vi "SC2 Host.vi"() -> ()   [LabVIEW 2015]
uses:
  SC2 states.ctl
  Interface states.ctl
panel:
  out "Change Complete?":bool
  out "Motor status":bool
  out "Current Sample":u8
  in  "Random Change":bool
  in  "stop":bool
  out "error out":errorcluster
  in  "error in (no error)":errorcluster
  in  "Encoder Offset":i16=-1021
  in  "Requested Sample":u8
  out "SC2 State Control":T1=enum."wait"
  out "Raw Encoder":bool[](array[boolean])
  out "Converted Encoder":bool[](array[boolean])
  out "Encoder Position":i32
  out "Motor Done?":bool
  in  "Start Sample Change":bool
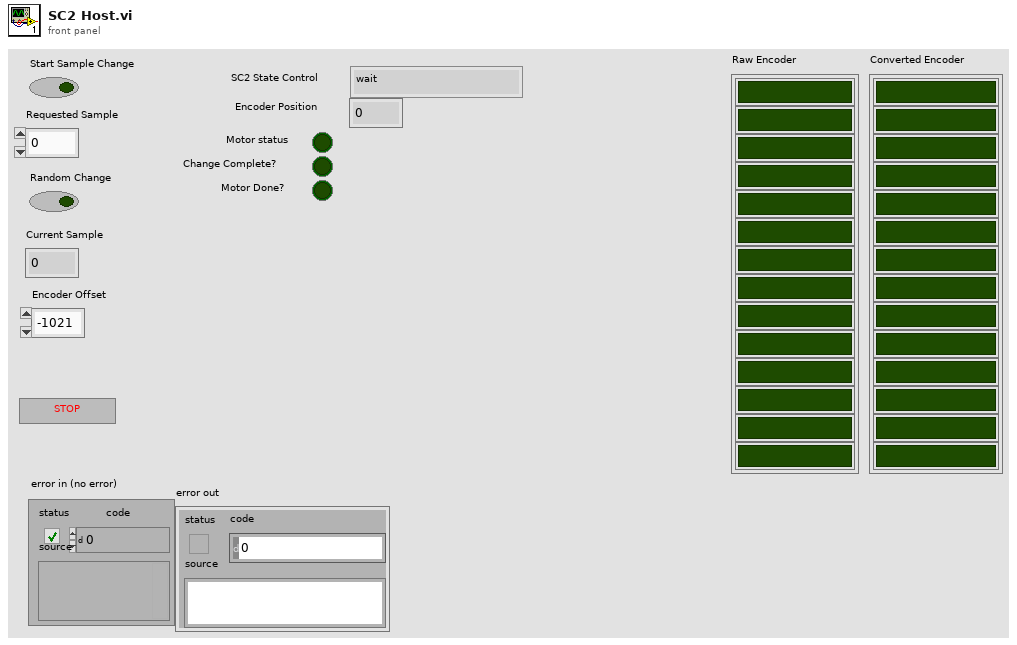
[diagram p1: front panel]
types:
  T1 = typedef "SC2 states.ctl" = enum16{"initialize", "wait", "check position", "rotate wheel", "rotate complete"}
  T2 = typedef "Interface states.ctl" = enum16{"Initialization", "Wait", "start wheel change", "Shutdown"}
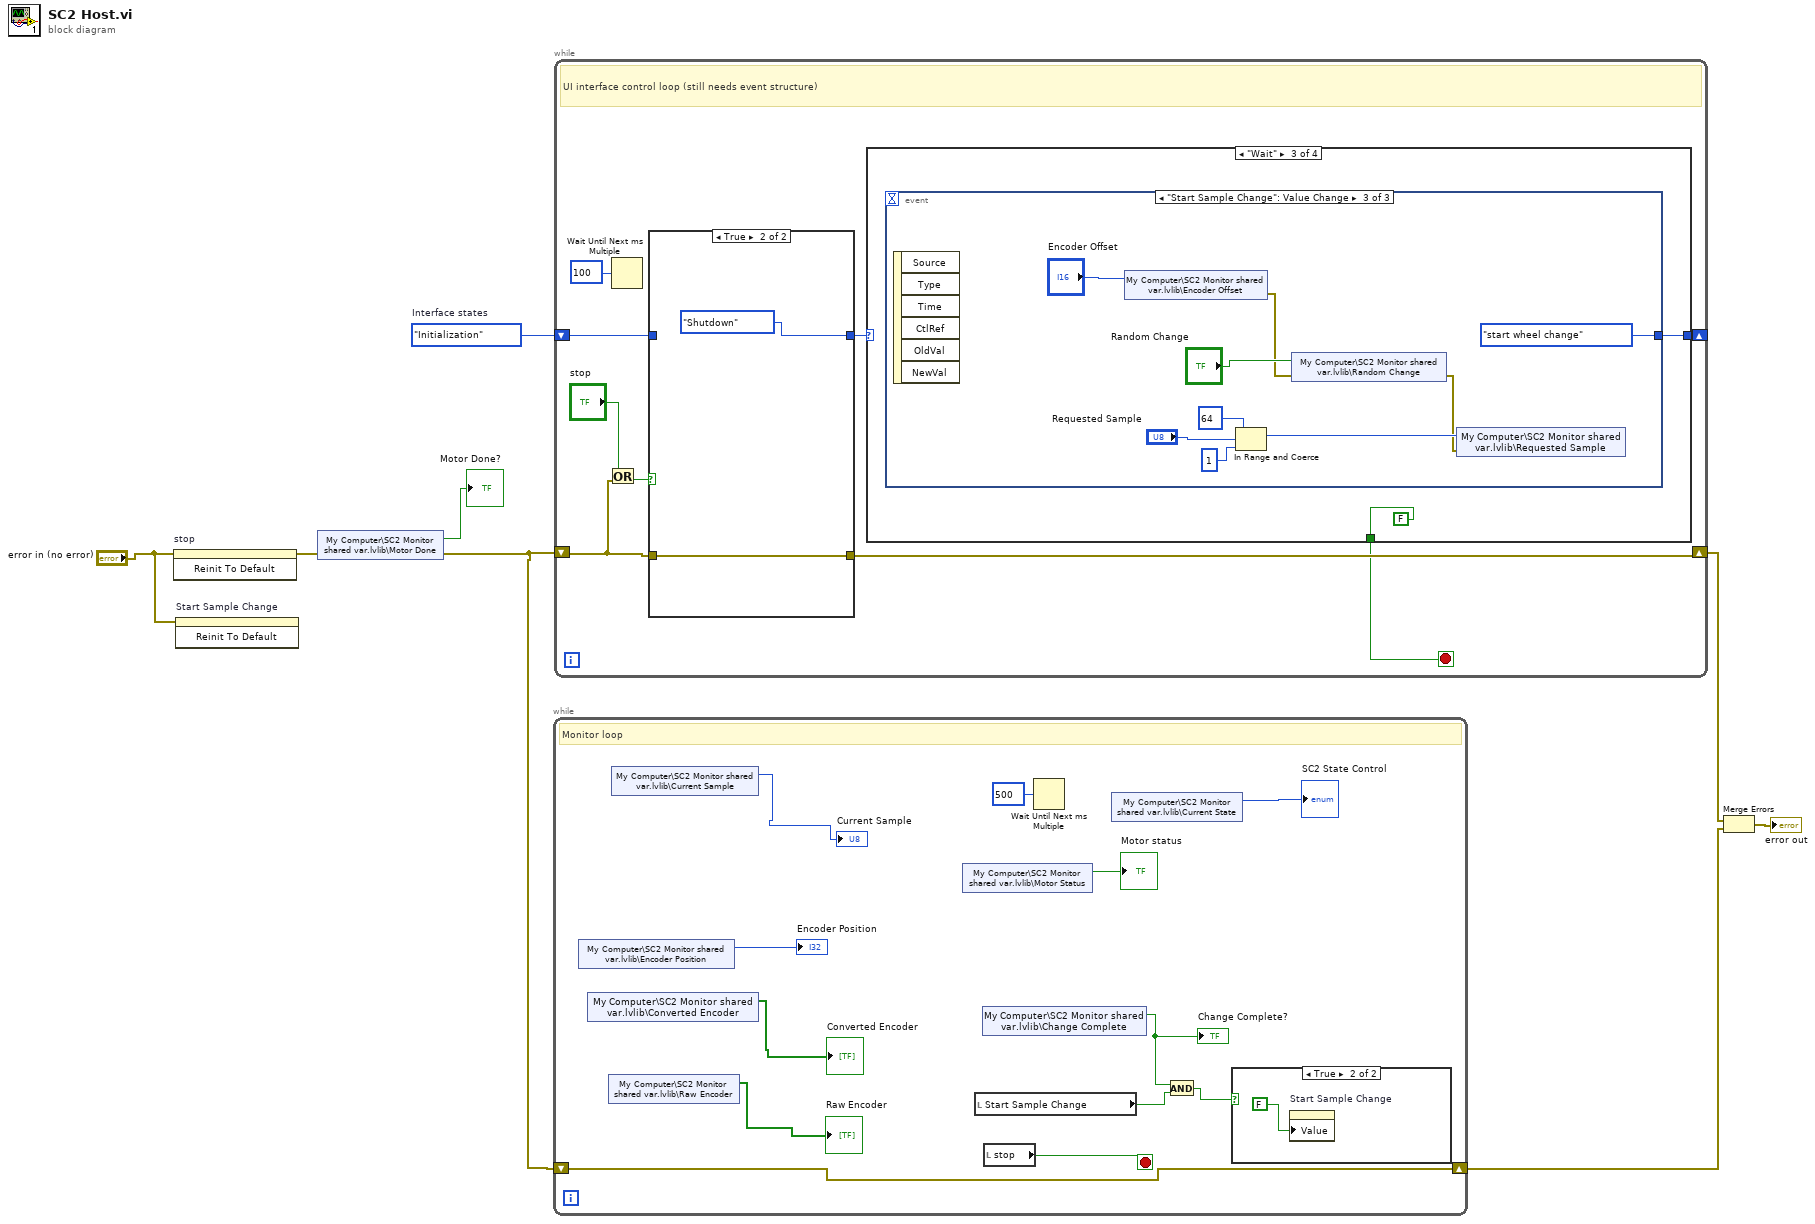
[diagram p0: block diagram]
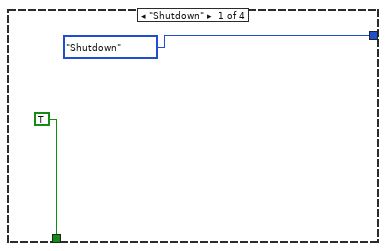
[diagram p4: hidden frame]
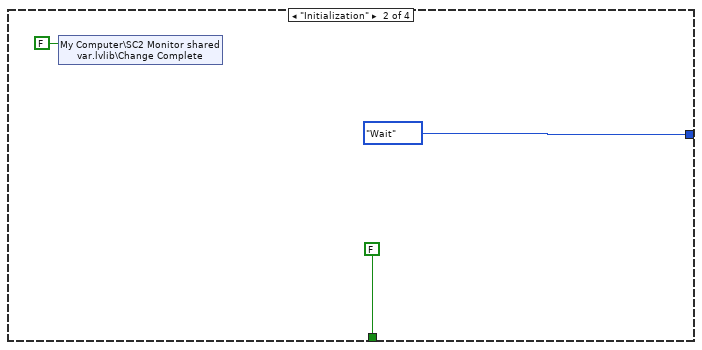
[diagram p5: hidden frame]
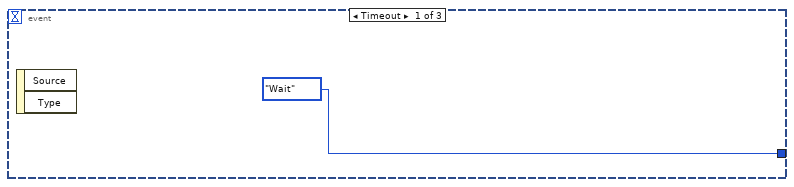
[diagram p6: hidden frame]
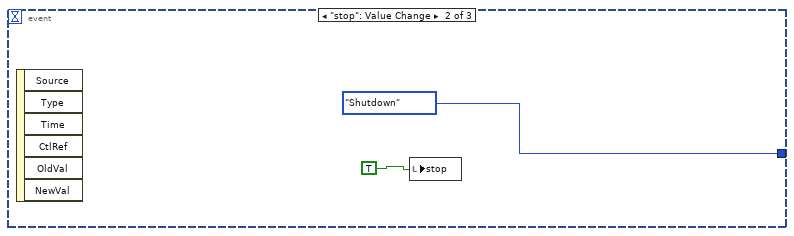
[diagram p7: hidden frame]
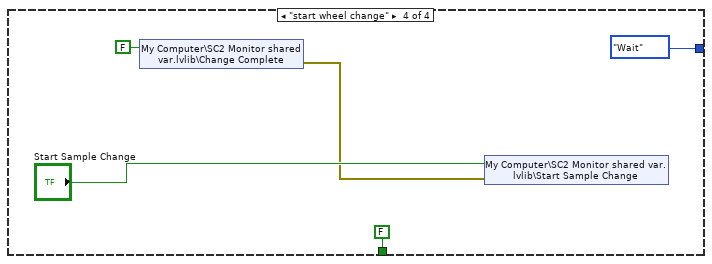
[diagram p8: hidden frame]
diagram:
  w3 = Interface_states."Initialization"  # Interface states
  n1 = invoke on="stop" class="Bool (strict)" method="Reinit To Default"(error in="error in (no error)") -> (error out=w1:errorcluster)  [unwired: 2 in, 2 out]
  n2 = invoke on="Start Sample Change" class="Bool (strict)" method="Reinit To Default"(error in="error in (no error)") -> ()  [unwired: 2 in, 3 out]
  n3 = shared-variable "My Computer\\SC2 Monitor shared var.lvlib\\Motor Done"(error in=w1) -> (→"Motor Done?":bool, error out=w4:errorcluster)
  n4 = while {
    shift-right: [w19] -> w6
    shift-left: w4 -> [w19]
    stop <- w18 stop-if-true
    # "Monitor loop"
    n5 = shared-variable "My Computer\\SC2 Monitor shared var.lvlib\\Encoder Position"() -> (→"Encoder Position":i32)  [unwired: 1 in, 1 out]
    n6 = shared-variable "My Computer\\SC2 Monitor shared var.lvlib\\Converted Encoder"() -> (→"Converted Encoder":bool[])  [unwired: 1 in, 1 out]
    n7 = shared-variable "My Computer\\SC2 Monitor shared var.lvlib\\Raw Encoder"() -> (→"Raw Encoder":bool[])  [unwired: 1 in, 1 out]
    n8 = shared-variable "My Computer\\SC2 Monitor shared var.lvlib\\Current Sample"() -> (→"Current Sample":u8)  [unwired: 1 in, 1 out]
    n9 = shared-variable "My Computer\\SC2 Monitor shared var.lvlib\\Motor Status"() -> (→"Motor status":bool)  [unwired: 1 in, 1 out]
    n10 = local read "Start Sample Change"() -> (w16:bool)
    n11 = shared-variable "My Computer\\SC2 Monitor shared var.lvlib\\Change Complete"() -> (w12:bool)  [unwired: 1 in, 1 out]
    "Change Complete?" <- w12
    n12 = local read "stop"() -> (w18:bool)
    n13 = Wait Until Next ms Multiple(millisecond multiple=u32 500) -> ()  [unwired: 1 out]
    n14 = shared-variable "My Computer\\SC2 Monitor shared var.lvlib\\Current State"() -> (→"SC2 State Control":u16)  [unwired: 1 in, 1 out]
    n15 = And(x=w12, y=w16) -> (x .and. y?=w17:bool)
    n16 = case shown="True" w17 {
      frame False {
      }
      frame True {
        n17 = property on="Start Sample Change" class="Bool (strict)"("Value"=FALSE ("Start Sample Change")) -> ()  [unwired: 2 in, 2 out]
      }
    }
  }
  n18 = while {
    shift-right: [w27] -> w5
    shift-left: w4 -> [w23]
    shift-right: [w29] -> _
    shift-left: w3 -> [w25]
    stop <- w22 stop-if-true
    # "UI interface control loop (still needs event structure)"
    n19 = Or(x="stop", y=w23) -> (x .or. y?=w24:bool)
    n20 = Wait Until Next ms Multiple(millisecond multiple=u32 100) -> ()  [unwired: 1 out]
    n21 = case shown="True" w24 {
      tunnel: w23 -> [w32 w33]
      tunnel: [w32 w33] -> w27
      tunnel: [w31 Interface_states."Shutdown" ("Interface states")] -> w26
      tunnel: w25 -> [w31 _]
      frame False {
      }
      frame True {
      }
    }
    n22 = case shown="\"Wait\"" w26 {
      tunnel: [Interface_states."Shutdown" ("Interface states") Interface_states."Wait" ("Interface states") w40 Interface_states."Wait" ("Interface states")] -> w29
      tunnel: [TRUE FALSE FALSE FALSE] -> w22
      frame "Shutdown" {
      }
      frame "Initialization" {
        n23 = shared-variable "My Computer\\SC2 Monitor shared var.lvlib\\Change Complete"(FALSE ("SC2 Change Complete")) -> ()  [unwired: 1 in, 1 out]
      }
      frame "Wait" {
        n24 = event shown="[2] \"Start Sample Change\": Value Change" {
          selector: _ -> [_ _ _]
          dyn-events: _ -> [_ _ _]
          timeout: _ -> [_ _ _]
          tunnel: [Interface_states."Wait" ("Interface states") Interface_states."Shutdown" ("Interface states") Interface_states."start wheel change" ("Interface states")] -> w40
          event Timeout {
            n25 = event-data() -> ()  [unwired: 1 in, 2 out]
          }
          event "stop": Value Change {
            n26 = event-data() -> ()  [unwired: 1 in, 6 out]
            n27 = local write "stop"(TRUE ("stop")) -> ()
          }
          event "Start Sample Change": Value Change {
            n28 = event-data() -> ()  [unwired: 1 in, 6 out]
            n29 = shared-variable "My Computer\\SC2 Monitor shared var.lvlib\\Encoder Offset"("Encoder Offset") -> (error out=w45:errorcluster)  [unwired: 1 in]
            n30 = In Range and Coerce(upper limit=u8 64, x="Requested Sample", lower limit=u8 1) -> (coerced(x)=w51:u8)  [unwired: 1 out]
            n31 = shared-variable "My Computer\\SC2 Monitor shared var.lvlib\\Random Change"("Random Change", error in=w45) -> (error out=w47:errorcluster)
            n32 = shared-variable "My Computer\\SC2 Monitor shared var.lvlib\\Requested Sample"(w51, error in=w47) -> ()  [unwired: 1 out]
          }
        }
      }
      frame "start wheel change" {
        n33 = shared-variable "My Computer\\SC2 Monitor shared var.lvlib\\Change Complete"(FALSE ("SC2 Change Complete")) -> (error out=w54:errorcluster)  [unwired: 1 in]
        n34 = shared-variable "My Computer\\SC2 Monitor shared var.lvlib\\Start Sample Change"("Start Sample Change", error in=w54) -> ()  [unwired: 1 out]
      }
    }
  }
  n35 = Merge Errors(w5, w6) -> (→"error out":errorcluster)
